vi "Delete Laplacian 64f.vi"(8 "Error In":errorcluster, 11 "Laplacian Object":T1 {"Laplacian Out"."Dimension"."Width" min=1; "Laplacian Out"."Dimension"."Height" min=1; "Laplacian Out"."Dimension"."Depth" min=1}) -> (0 "Error Out":errorcluster)   [LabVIEW 2012, in "OpenCLV x64.lvlib"]
doc: "Deletes the Laplacian Object and all associated memory."
uses:
  OpenCLV x64.lvlib
  Controls/Laplacian Object.ctl
  Controls/Device ID.ctl
  Controls/Program Handle.ctl
  Controls/Memory Object.ctl
  Controls/Memory ID.ctl
  User Controls/Array Dimensions.ctl
  Controls/Memory Type.ctl
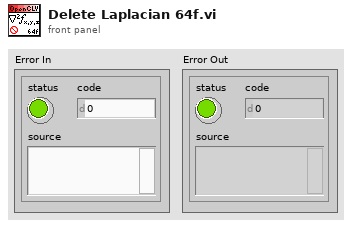
[diagram p1: front panel]
types:
  T1 = typedef "OpenCLV x64.lvlib/Laplacian Object.ctl" = cluster{"Device Out":T2, "Program Handle":T3, "Laplacian Out":T4}
  T2 = typedef "OpenCLV x64.lvlib/Device ID.ctl" = u64
  T3 = typedef "OpenCLV x64.lvlib/Program Handle.ctl" = u64
  T4 = typedef "OpenCLV x64.lvlib/Memory Object.ctl" = cluster{"Device ID":T2, "Memeroy ID":T5, "Dimension":T6, "Memory Type":T7}
  T5 = typedef "OpenCLV x64.lvlib/Memory ID.ctl" = u64
  T6 = typedef "Array Dimensions.ctl" = cluster{"Depth":u64, "Height":u64, "Width":u64}
  T7 = typedef "OpenCLV x64.lvlib/Memory Type.ctl" = enum16{"32f", "u8", "i8", "u16", "i16", "u32", "i32", "64f"}
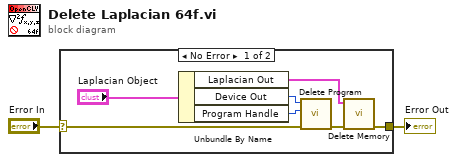
[diagram p0: block diagram]
diagram:
  n1 = case shown="No Error" "Error In" {
    selector: "Error In" -> [w8 w10]
    tunnel: [w5 w10] -> w1
    frame No Error {
      n2 = Unbundle By Name("Laplacian Object") -> ("Laplacian Out"=w3:T4, "Device Out"=w4:T2, "Program Handle"=w9:T3)
      n3 = call "Delete Program.vi"("Error In"=w8, "Program In"=w9, "Device ID"=w4) -> ("Error Out"=w7:errorcluster)  [unwired: 8 in]
      n4 = call "Delete Memory.vi"("Error In"=w7, "Memory Object In"=w3) -> ("Error Out"=w5:errorcluster)  [unwired: 8 in, 1 out]
    }
    frame Error {
    }
  }
  "Error Out" <- w1
